vi "FindMessages.vi"(7 "ConcreteActor":refnum<class "ConcreteActor.lvclass">) -> (3 "Messages":T1)   [LabVIEW 2020, in "jettl.lvlib" / "Base.lvlib" / "ConcreteActor.lvclass"]
uses:
  ConcreteActor.lvclass
  Message/Message.lvclass
  ConcreteActor.lvclass/ConcreteActor.ctl
  jettl.lvlib
  MessageSet.ctl
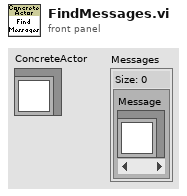
[diagram p1: front panel]
types:
  T1 = typedef "jettl.lvlib/MessageSet.ctl" = set{refnum<class "Message.lvclass">}
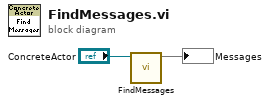
[diagram p0: block diagram]
diagram:
  n1 = call "FindMessages.vi"("ConcreteActor.lvclass"="ConcreteActor") -> ("Messages"=→"Messages":T1)  [unwired: 10 in]
